vi "Zaber A Series Move.vi"() -> ()   [LabVIEW 2015]
doc: "This beginner example shows the Move VI, which allows the user to move devices based on real-world units easily."
uses:
  Zaber A Series.lvlib
panel:
  in  "Units (0: microsteps)":u16(ring) items=["microsteps", "microns", "millimeters", "inches", "degrees"]
  in  "Movement Type (0: relative)":u16(ring) items=["relative", "absolute"]
  in  "Device and Axis":string
  in  "Microstep Size (0)":dbl
  in  "Move Distance (0)":dbl format="%#_6f"
  in  "VISA resource name":refnum<visa-resource-name>
  # "(c) 2017 Zaber Technologies.  ALL RIGHTS RESERVED."
  # "This example shows how you can use the Move VI to make movements easily.\nThe Move VI allows you to use real world units while moving the stage. This is\nuseful because typically you would send movement commands with microstep\nvalues and make conversions to see how it relates to real units. To use these\nunits (except microsteps) make sure to input the Microstep Size before running.\nvalue can be found on spec page for the product on www.zaber.com."
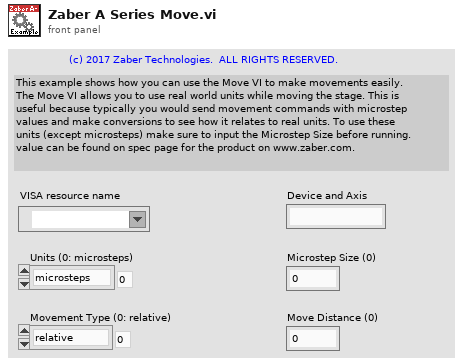
[diagram p1: front panel]
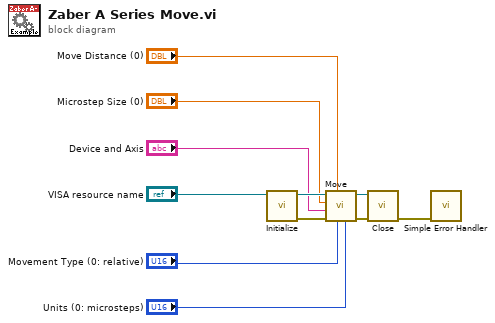
[diagram p0: block diagram]
diagram:
  n1 = call "Initialize.vi"("VISA resource name"="VISA resource name") -> ("error out"=w8:errorcluster, "VISA resource name out"=w10:refnum<visa-resource-name>)  [unwired: 9 in]
  n2 = call "Move.vi"("Units (0: microsteps)"="Units (0: microsteps)", "Movement Type (0: relative)"="Movement Type (0: relative)", "Move Distance (0)"="Move Distance (0)", "error in (no error)"=w8, "Device and Axis"="Device and Axis", "Microstep Size (0)"="Microstep Size (0)", "VISA resource name"=w10) -> ("error out"=w7:errorcluster, "VISA resource name out"=w9:refnum<visa-resource-name>)  [unwired: 3 in]
  n3 = call "Close.vi"("error in (no error)"=w7, "VISA resource name"=w9) -> ("error out"=w6:errorcluster)  [unwired: 9 in]
  n4 = call <vilib>:"Simple Error Handler.vi"("error in (no error)"=w6) -> ()  [unwired: 4 in, 5 out]
